vi "CMDcontrolKNRm.vi"(8 "cnt":i32, 10 "prefed":dbl, 11 "Tcmd":dbl) -> (0 "itrflg":i32, 2 "Ocmd":dbl, 3 "Tcmd":dbl)   [LabVIEW 2013]
uses:
  Global_KNRm.vi
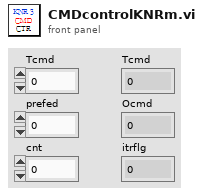
[diagram p1: front panel]
types:
  T1 = cluster{"Nacc":i32, "deg":dbl, "cnt":i32, "Tacc":dbl, "Lest":dbl, "Ocmd":dbl, "Nc":i32, "Lmin":dbl, "Tcmd":dbl, "Tc":dbl, "Type":i32, "itrflg":i32}
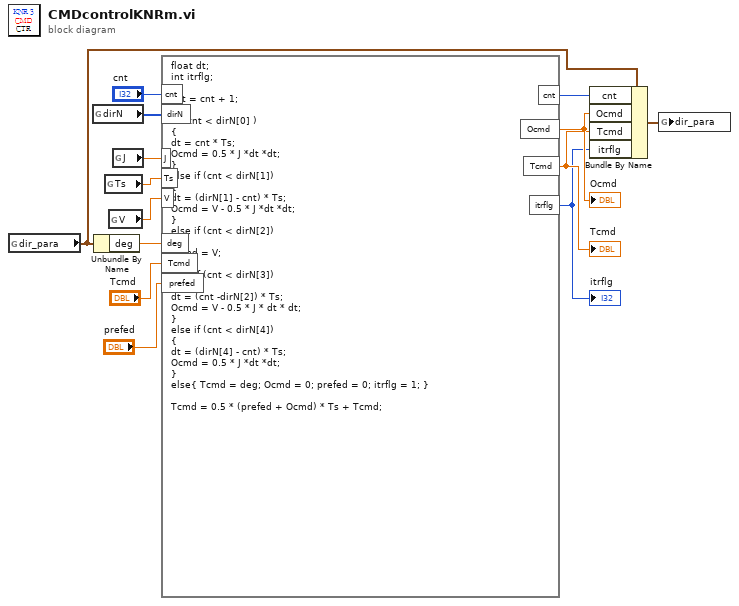
[diagram p0: block diagram]
diagram:
  n1 = global read "Global_KNRm.vi" "dir_para"() -> (w6:T1)
  n2 = global read "Global_KNRm.vi" "dirN"() -> (w13:i32[])
  n3 = Unbundle By Name(w6) -> ("deg"=w8:dbl)
  n4 = global read "Global_KNRm.vi" "Ts"() -> (w11:dbl)
  n5 = global read "Global_KNRm.vi" "V"() -> (w10:dbl)
  n6 = global read "Global_KNRm.vi" "J"() -> (w12:dbl)
  n7 = formula code="float dt;\nint itrflg;\n\ncnt = cnt + 1;\n\nif ( cnt < dirN[0] )\n{\ndt = cnt * Ts; \nOcmd = 0.5 * J *dt *dt;\n}\nelse if (cnt < dirN[1])\n{\ndt = (dirN[1] - cnt) * Ts;\nOcmd = V - 0.5 * J *dt *dt;\n}\nelse if (cnt < dirN[2])\n{\nOcmd = V;\n}\nelse if (cnt < dirN[3])\n{\ndt = (cnt -dirN[2]) * Ts;\nOcmd = V - 0.5 * J * dt * dt;\n}\nelse if (cnt < dirN[4])\n{\ndt = (dirN[4] - cnt) * Ts;\nOcmd = 0.5 * J *dt *dt;\n}\nelse{ Tcmd = deg; Ocmd = 0; prefed = 0; itrflg = 1; }\n\nTcmd = 0.5 * (prefed + Ocmd) * Ts + Tcmd;"("cnt"="cnt", "dirN"=w13, "J"=w12, "Ts"=w11, "V"=w10, "deg"=w8, "Tcmd"="Tcmd", "prefed"="prefed") -> ("cnt"=w5:i32, "Ocmd"=w4:dbl, "Tcmd"=w3:dbl, "itrflg"=w2:i32)
  "Tcmd" <- w3
  "Ocmd" <- w4
  "itrflg" <- w2
  n8 = Bundle By Name(cluster=w6, "cnt"=w5, "Ocmd"=w4, "Tcmd"=w3, "itrflg"=w2) -> (w1:T1)
  n9 = global write "Global_KNRm.vi" "dir_para"(w1) -> ()
